vi "Main.vi"() -> ()   [LabVIEW 2020]
doc: "Retrieves average CPU temp, if available. No warranty, use it at your own risk.\n\n© Aitor Solar, 2019.\nContact: aitor.solar@gmail.com"
uses:
  <vilib>/Platform/TimedLoop/XDataNode/timing_clust.ctl
  <vilib>/Platform/TimedLoop/XDataNode/nitl_modes.ctl
  <vilib>/Platform/TimedLoop/XDataNode/wakeup.ctl
  <vilib>/platform/TimedLoop/XDataNode/XDataNode.xnode
  <vilib>/Platform/TimedLoop/XDataNode/XDNodeRunTimeDep.lvlib
panel:
  out "Output Filename":path
  in  "Output Directory":path=path "C:/Users/Josh/Desktop/code/CVB/Config/generated_data"
  in  "Create New File":bool=TRUE
  in  "Thermocouple selector":enum16{"High Accuracy", "High Speed"}(ring)
  out "Waveform Chart":dynamicdata(graph)
  in  "stop":bool
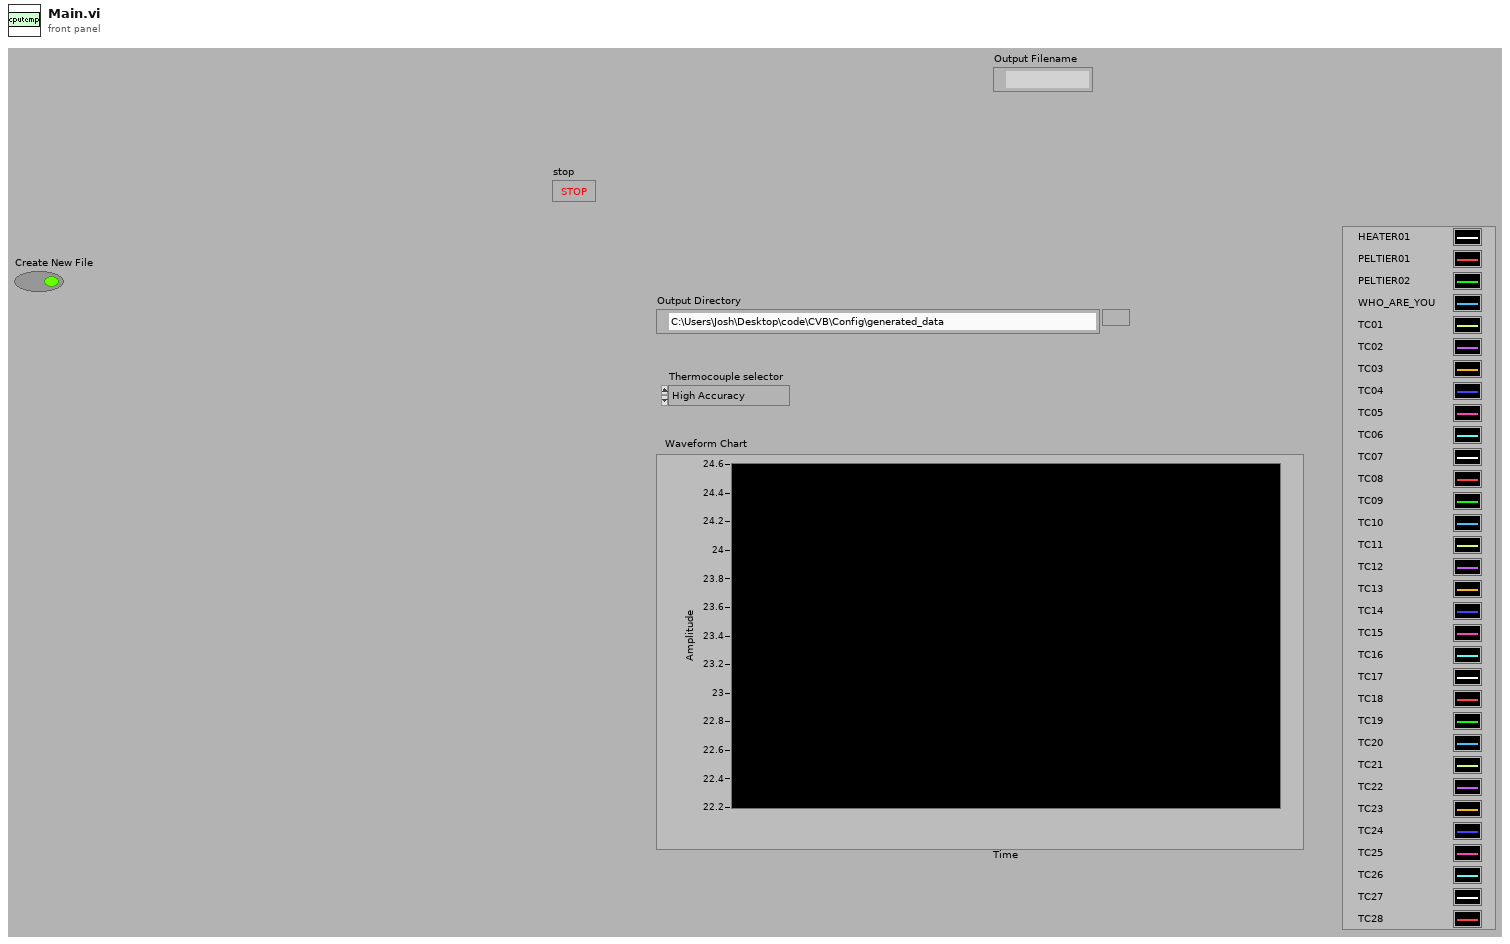
[diagram p1: front panel]
types:
  T1 = typedef "XDNodeRunTimeDep.lvlib/timing_clust.ctl" = cluster{"Expected End [f-1]":u64, "Actual End [f-1]":u64, "Finished Late? [f-1]":bool, "Expected End [i-1]":u64, "Actual End [i-1]":u64, "Finished Late? [i-1]":bool, "Expected Start [i]":u64, "Actual Start [i]":u64, "Expected Start [f]":u64, "Actual Start [f]":u64, "Source Name":string, "Structure Name":string, "Period":i64, "Deadline":i64, "Offset":i64, "Start":i64, "Priority":i32, "Timeout":i32, "Mode":T2, "Wakeup Reason":T3, "Error":errorcluster, "Source Type":string, "Secondary Source Type":string, "Global End Time":u64, "Global Start Time":u64, "Frame Duration":u64, "Iteration Duration":u64, "Assigned CPU":i32, "I/O Scan Engine Mode":u32}
  T2 = typedef "XDNodeRunTimeDep.lvlib/nitl_modes.ctl" = enum32{"No Change", "Process missed periods, maintain original phase", "Discard missed periods, maintain original phase", "Process missed periods, ignore original phase", "Discard missed periods, ignore original phase"}
  T3 = typedef "XDNodeRunTimeDep.lvlib/wakeup.ctl" = enum32{"Normal", "Aborted", "Asynchronous wakeup", "Timing source error", "Timed loop error", "Timeout"}
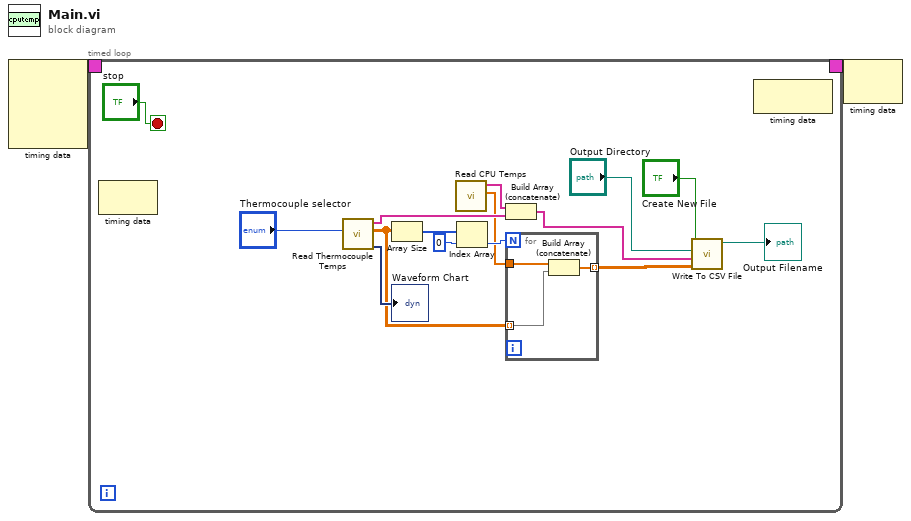
[diagram p0: block diagram]
diagram:
  n1 = node-c288() -> (w2:T1)  [unwired: 4 in]
  n2 = timed-loop {
    timing: w2 -> [_]
    timing-out: [_] -> w1
    stop <- "stop" stop-if-true
    n3 = node-c288() -> ()  [unwired: 1 in, 1 out]
    n4 = call "Read Thermocouple Temps.vi"("Thermocouple selector"="Thermocouple selector") -> ("data"=→"Waveform Chart":dynamicdata, "Values"=w8:dbl[][], "Names"=w13:string[])  [unwired: 8 in]
    n5 = Array Size(array=w8) -> (size(s)=w12:i32[])
    n6 = call "Read CPU Temps.vi"() -> ("Termperatures"=w9:dbl[], "Names"=w14:string[])  [unwired: 9 in, 1 out]
    n7 = Index Array(array=w12, index=0) -> (element=w10:i32)
    n8 = Build Array (concatenate)(w14, w13) -> (w6:string[])
    n9 = for {
      N: w10 -> [_]
      tunnel: w8 -> [w20] mode=indexing
      tunnel: w9 -> [w19]
      tunnel: [w18] -> w5 mode=indexing
      n10 = Build Array (concatenate)(w19, w20) -> (w18:dbl[])
    }
    n11 = call "Write To CSV File.vi"("Values"=w5, "Names"=w6, "Output Directory"="Output Directory", "Create New File"="Create New File") -> ("Output Filename"=→"Output Filename":path)  [unwired: 7 in]
    n12 = node-c288() -> ()  [unwired: 1 in, 1 out]
  }
  n13 = node-c288(w1) -> ()  [unwired: 1 out]
